vi "Hahn 3 pi vs no pi contrast Pulse Sequence Generator.vi"(0 "N Loop":i32=10000, 1 "Rabi Freq":dbl=7000000.0, 3 "Tau Min":dbl=2e-08, 5 "AOM Pulse length":dbl=2.5e-06, 7 "AOM Rest time":dbl=1e-06, 9 "Signal Delay":dbl=6e-07, 10 "Tau No. Steps":i32=20, 11 "APD signal width":dbl=5e-07, 12 "MW Delay":dbl, 14 "Tau Max":dbl=0.001, 15 "type":u16(ring)=1 items=["Linear", "Logarithmic"]) -> (4 "Pulse Sequence":T1(array[cluster]), 6 "Tau":dbl[](array[numeric]))   [LabVIEW 2012]
uses:
  <vilib>/Analysis/1siggen.llb/Ramp Pattern by Samples.vi
  <vilib>/Analysis/NI_AALBase.lvlib
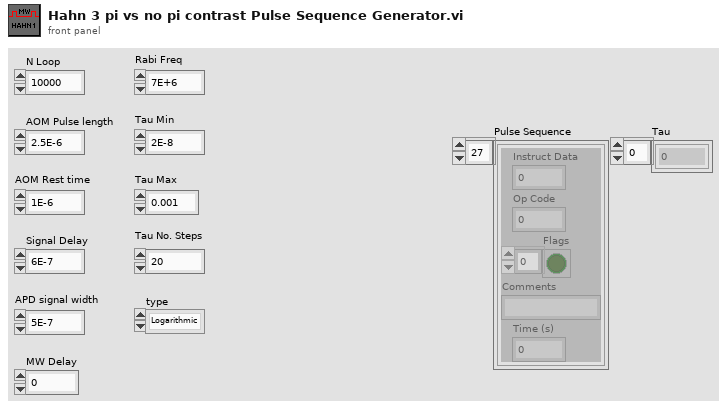
[diagram p1: front panel]
types:
  T1 = cluster{"Instruct Data":i32, "Op Code":i32, "Flags":bool[], "Comments":string, "Time (s)":dbl}[]
  T2 = cluster{"Instruct Data":i32, "Op Code":i32, "Flags":bool[], "Comments":string, "Time (s)":dbl}
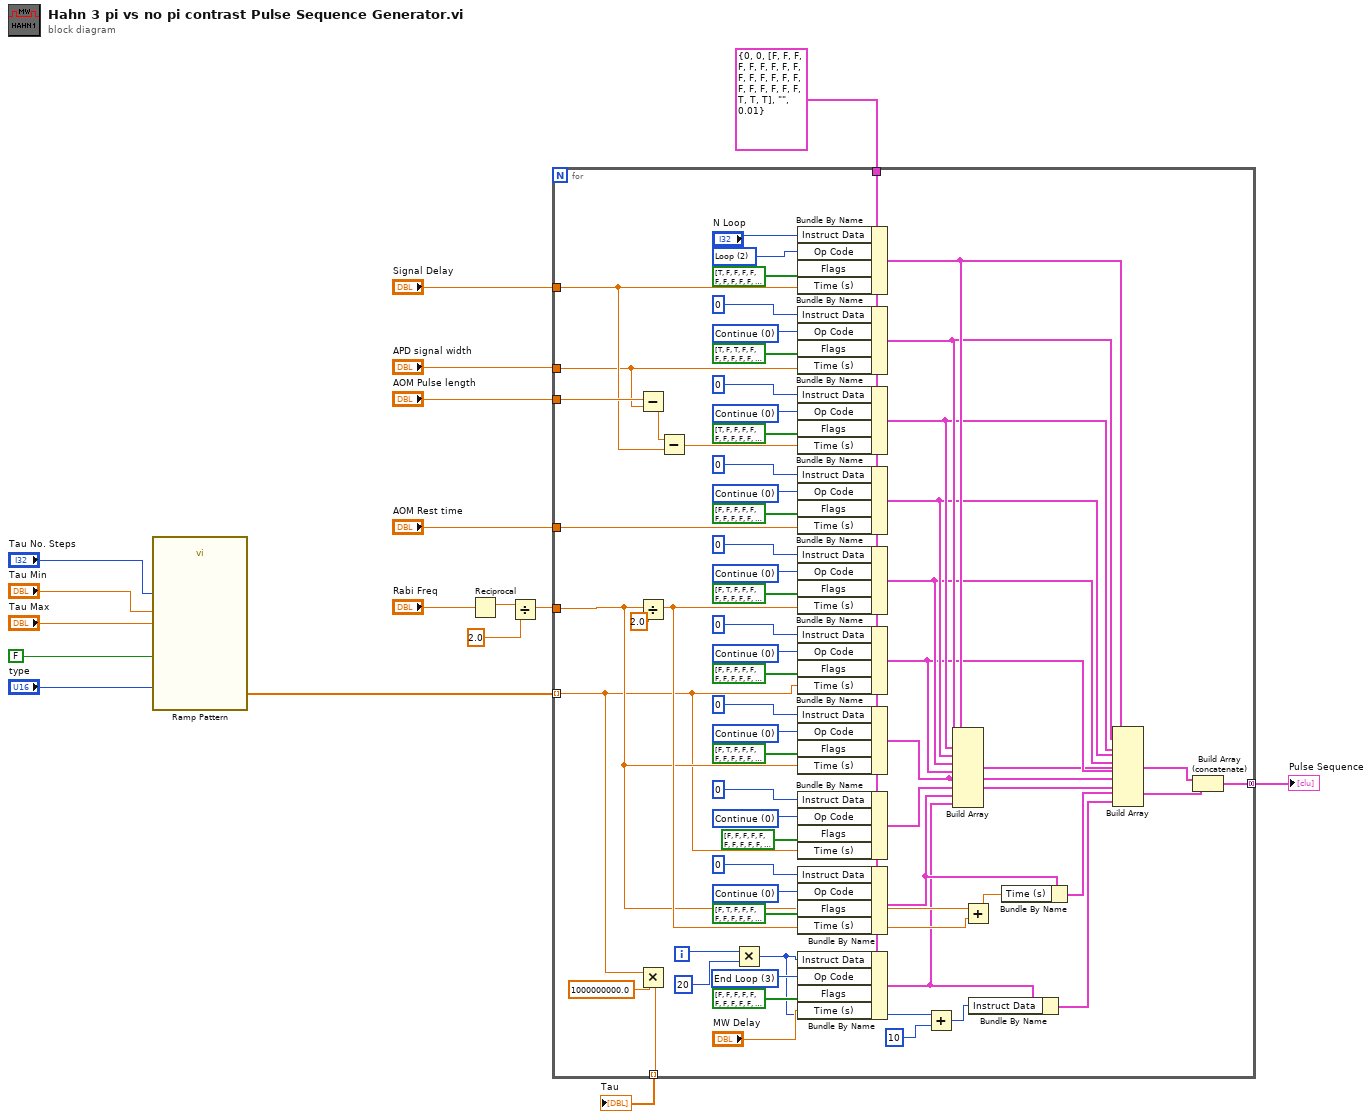
[diagram p0: block diagram]
diagram:
  n1 = call-poly <vilib>:"Ramp Pattern.vi"("type"="type", "exclude end?"=FALSE, "start"="Tau Min", "end"="Tau Max", "samples"="Tau No. Steps") -> ("Ramp Pattern"=w3:dbl[])  [unwired: 5 in, 1 out]
  n2 = Reciprocal(x="Rabi Freq") -> (1/x=w6:dbl)
  n3 = Divide(x=w6, y=2.0) -> (x/y=w7:dbl)
  n4 = for {
    tunnel: "Signal Delay" -> [w63]
    tunnel: "APD signal width" -> [w62]
    tunnel: "AOM Pulse length" -> [w73]
    tunnel: "AOM Rest time" -> [w60]
    tunnel: w7 -> [w30]
    tunnel: w3 -> [w20] mode=indexing
    tunnel: T2 {"Instruct Data"=0, "Op Code"=0, "Flags"=[FALSE, FALSE, FALSE, FALSE, FALSE, FALSE, FALSE, FALSE, FALSE, FALSE, FALSE, FALSE, FALSE, FALSE, FALSE, FALSE, FALSE, FALSE, FALSE, FALSE, FALSE, TRUE, TRUE, TRUE], "Comments"="", "Time (s)"=0.01} ("PB Inst 2") -> [w19]
    tunnel: [w57] -> w1 mode=concatenating
    tunnel: [w54] -> w2 mode=indexing
    i -> [w59]
    w41 = 3 items=["Continue", "Stop", "Loop", "End Loop", "JSR", "RTS", "Branch", "Long Delay", "Wait"] ("Op Code")
    w45 = 0 items=["Continue", "Stop", "Loop", "End Loop", "JSR", "RTS", "Branch", "Long Delay", "Wait"] ("Op Code")
    w48 = 0 items=["Continue", "Stop", "Loop", "End Loop", "JSR", "RTS", "Branch", "Long Delay", "Wait"] ("Op Code")
    w51 = 0 items=["Continue", "Stop", "Loop", "End Loop", "JSR", "RTS", "Branch", "Long Delay", "Wait"] ("Op Code")
    w65 = 0 items=["Continue", "Stop", "Loop", "End Loop", "JSR", "RTS", "Branch", "Long Delay", "Wait"] ("Op Code")
    w68 = 0 items=["Continue", "Stop", "Loop", "End Loop", "JSR", "RTS", "Branch", "Long Delay", "Wait"] ("Op Code")
    w70 = 0 items=["Continue", "Stop", "Loop", "End Loop", "JSR", "RTS", "Branch", "Long Delay", "Wait"] ("Op Code")
    w75 = 0 items=["Continue", "Stop", "Loop", "End Loop", "JSR", "RTS", "Branch", "Long Delay", "Wait"] ("Op Code")
    w78 = 0 items=["Continue", "Stop", "Loop", "End Loop", "JSR", "RTS", "Branch", "Long Delay", "Wait"] ("Op Code")
    w80 = 2 items=["Continue", "Stop", "Loop", "End Loop", "JSR", "RTS", "Branch", "Long Delay", "Wait"] ("Op Code")
    n5 = Subtract(x=w73, y=w62) -> (x-y=w72:dbl)
    n6 = Divide(x=w30, y=2.0) -> (x/y=w31:dbl)
    n7 = Multiply(x=w20, y=1000000000.0) -> (x*y=w54:dbl)
    n8 = Subtract(x=w72, y=w63) -> (x-y=w61:dbl)
    n9 = Multiply(x=w59, y=20) -> (x*y=w26:i32)
    n10 = Bundle By Name(cluster=w19, "Instruct Data"="N Loop", "Op Code"=w80, "Flags"=bool[] [TRUE, FALSE, FALSE, FALSE, FALSE, FALSE, FALSE, FALSE, FALSE, FALSE, FALSE, FALSE, FALSE, FALSE, FALSE, FALSE, FALSE, FALSE, FALSE, FALSE, FALSE, TRUE, TRUE, TRUE], "Time (s)"=w63) -> (w39:T2)
    n11 = Bundle By Name(cluster=w19, "Instruct Data"=0, "Op Code"=w78, "Flags"=bool[] [TRUE, FALSE, TRUE, FALSE, FALSE, FALSE, FALSE, FALSE, FALSE, FALSE, FALSE, FALSE, FALSE, FALSE, FALSE, FALSE, FALSE, FALSE, FALSE, FALSE, FALSE, TRUE, TRUE, TRUE], "Time (s)"=w62) -> (w38:T2)
    n12 = Bundle By Name(cluster=w19, "Instruct Data"=0, "Op Code"=w75, "Flags"=bool[] [TRUE, FALSE, FALSE, FALSE, FALSE, FALSE, FALSE, FALSE, FALSE, FALSE, FALSE, FALSE, FALSE, FALSE, FALSE, FALSE, FALSE, FALSE, FALSE, FALSE, FALSE, TRUE, TRUE, TRUE], "Time (s)"=w61) -> (w37:T2)
    n13 = Bundle By Name(cluster=w19, "Instruct Data"=0, "Op Code"=w70, "Flags"=bool[] [FALSE, FALSE, FALSE, FALSE, FALSE, FALSE, FALSE, FALSE, FALSE, FALSE, FALSE, FALSE, FALSE, FALSE, FALSE, FALSE, FALSE, FALSE, FALSE, FALSE, FALSE, TRUE, TRUE, TRUE], "Time (s)"=w60) -> (w36:T2)
    n14 = Bundle By Name(cluster=w19, "Instruct Data"=0, "Op Code"=w68, "Flags"=bool[] [FALSE, TRUE, FALSE, FALSE, FALSE, FALSE, FALSE, FALSE, FALSE, FALSE, FALSE, FALSE, FALSE, FALSE, FALSE, FALSE, FALSE, FALSE, FALSE, FALSE, FALSE, TRUE, TRUE, TRUE], "Time (s)"=w31) -> (w35:T2)
    n15 = Bundle By Name(cluster=w19, "Instruct Data"=0, "Op Code"=w65, "Flags"=bool[] [FALSE, FALSE, FALSE, FALSE, FALSE, FALSE, FALSE, FALSE, FALSE, FALSE, FALSE, FALSE, FALSE, FALSE, FALSE, FALSE, FALSE, FALSE, FALSE, FALSE, FALSE, TRUE, TRUE, TRUE], "Time (s)"=w20) -> (w34:T2)
    n16 = Bundle By Name(cluster=w19, "Instruct Data"=0, "Op Code"=w51, "Flags"=bool[] [FALSE, TRUE, FALSE, FALSE, FALSE, FALSE, FALSE, FALSE, FALSE, FALSE, FALSE, FALSE, FALSE, FALSE, FALSE, FALSE, FALSE, FALSE, FALSE, FALSE, FALSE, TRUE, TRUE, TRUE], "Time (s)"=w30) -> (w33:T2)
    n17 = Bundle By Name(cluster=w19, "Instruct Data"=0, "Op Code"=w48, "Flags"=bool[] [FALSE, FALSE, FALSE, FALSE, FALSE, FALSE, FALSE, FALSE, FALSE, FALSE, FALSE, FALSE, FALSE, FALSE, FALSE, FALSE, FALSE, FALSE, FALSE, FALSE, FALSE, TRUE, TRUE, TRUE], "Time (s)"=w20) -> (w18:T2)
    n18 = Bundle By Name(cluster=w19, "Instruct Data"=0, "Op Code"=w45, "Flags"=bool[] [FALSE, TRUE, FALSE, FALSE, FALSE, FALSE, FALSE, FALSE, FALSE, FALSE, FALSE, FALSE, FALSE, FALSE, FALSE, FALSE, FALSE, FALSE, FALSE, FALSE, FALSE, TRUE, TRUE, TRUE], "Time (s)"=w31) -> (w32:T2)
    n19 = Bundle By Name(cluster=w19, "Instruct Data"=w26, "Op Code"=w41, "Flags"=bool[] [FALSE, FALSE, FALSE, FALSE, FALSE, FALSE, FALSE, FALSE, FALSE, FALSE, FALSE, FALSE, FALSE, FALSE, FALSE, FALSE, FALSE, FALSE, FALSE, FALSE, FALSE, TRUE, TRUE, TRUE], "Time (s)"="MW Delay") -> (w27:T2)
    n20 = Add(x=w26, y=10) -> (x+y=w24:i32)
    n21 = Build Array(w39, w38, w37, w36, w35, w34, w33, w18, w32, w27) -> (w22:T1)
    n22 = Add(x=w30, y=w31) -> (x+y=w29:dbl)
    n23 = Bundle By Name(cluster=w27, "Instruct Data"=w24) -> (w23:T2)
    n24 = Bundle By Name(cluster=w32, "Time (s)"=w29) -> (w28:T2)
    n25 = Build Array(w39, w38, w37, w36, w35, w34, w33, w18, w28, w23) -> (w21:T1)
    n26 = Build Array (concatenate)(w22, w21) -> (w57:T1)
  }
  "Pulse Sequence" <- w1
  "Tau" <- w2
